vi "TiePie.Dev.DevGetType.vi"(8 "error in (no error) 2":errorcluster, 11 "GenHandle":T1) -> (0 "error out 2":errorcluster, 3 "deviceType":u32)   [LabVIEW 2014, in "LVTiePie.lvlib"]
uses:
  LVTiePie.lvlib
  TiePie.Gen.handle.ctl
  bin/libtiepie.dll
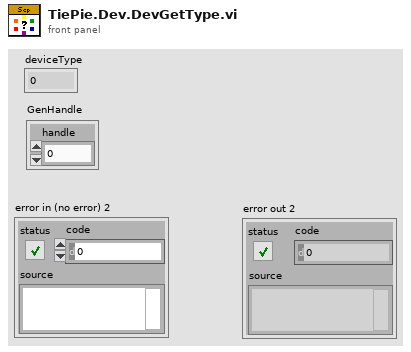
[diagram p1: front panel]
types:
  T1 = typedef "TiePie.Gen.handle.ctl" = cluster{"handle":u32}
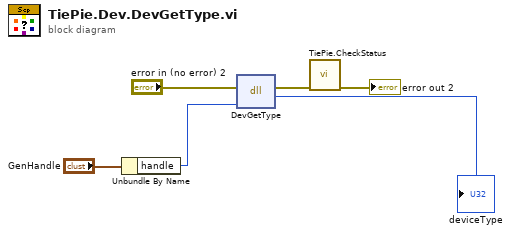
[diagram p0: block diagram]
diagram:
  n1 = Unbundle By Name("GenHandle") -> ("handle"=w5:u32)
  n2 = dll-call lib="C:/Users/mbirski/Desktop/PAN/LabVEW/Tie Pie/bin/libtiepie.dll" fn="DevGetType"(error in="error in (no error) 2", "handle"=w5) -> (error out=w3:errorcluster, "deviceType"=→"deviceType":u32)  [unwired: 3 in, 1 out]
  n3 = call "TiePie.CheckStatus.vi"("error in (no error)"=w3) -> ("error out"=→"error out 2":errorcluster)  [unwired: 10 in]
